vi "Meas_curr.vi"(8 "error in (no error)":errorcluster, 11 "Connection in":T1={"Baud"=9600, "Flow Ctl"=0, "COM port"="", "Parity"=0} {"Parity" items=["None", "Odd", "Even"]; "Flow Ctl" items=["None"]; "Baud" items=["4800"=4800, "9600"=9600, "19200"=19200, "38400"=38400]}) -> (0 "error out":errorcluster, 2 "Current":dbl, 3 "Connection out":T1={"Baud"=9600, "Flow Ctl"=0, "COM port"="", "Parity"=0} {"Parity" items=["None", "Odd", "Even"]; "Flow Ctl" items=["None"]; "Baud" items=["4800"=4800, "9600"=9600, "19200"=19200, "38400"=38400]})   [LabVIEW 2014, in "B&K Precision 9120 series.lvclass"]
uses:
  B&K Precision 9120 series.lvclass
  Serial_Config.ctl
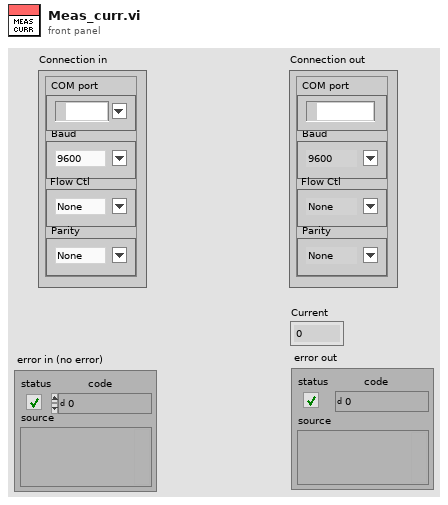
[diagram p1: front panel]
types:
  T1 = typedef "B&K Precision 9120 series.lvclass/Serial_Config.ctl" = cluster{"Baud":u32, "Flow Ctl":u16, "COM port":refnum<visa-resource-name>, "Parity":u16}
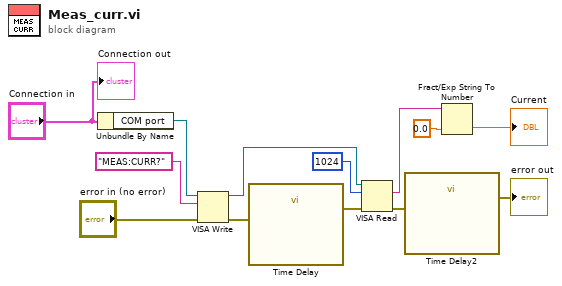
[diagram p0: block diagram]
diagram:
  n1 = Unbundle By Name("Connection in") -> ("COM port"=w6:refnum<visa-resource-name>)
  n2 = VISA Write(VISA resource name=w6, write buffer="MEAS:CURR?", error in (no error)="error in (no error)") -> (VISA resource name out=w12:refnum<visa-resource-name>, error out=w4:errorcluster)  [unwired: 1 out]
  n3 = call "Time Delay"("error in (no error)"=w4) -> ("error out"=w3:errorcluster)  [unwired: 10 in]
  n4 = VISA Read(VISA resource name=w12, byte count=u32 1024, error in (no error)=w3) -> (read buffer=w8:string, error out=w2:errorcluster)  [unwired: 2 out]
  n5 = call "Time Delay2"("error in (no error)"=w2) -> ("error out"=→"error out":errorcluster)  [unwired: 10 in]
  n6 = Fract/Exp String To Number(string=w8, default (0 dbl)=0.0 ("default (0 I32)")) -> (number=→"Current":dbl)  [unwired: 2 in, 1 out]
  "Connection out" <- "Connection in"
